vi "Word Report - Conditionally Formatted Table.vi"   [LabVIEW 2023]
doc: "This example shows how to format cells by their values in a Word document.\n\nThe VI sets the background color of the table cells to red if the cell value is greater than 90 and green if less than 10."
uses:
  <vilib>/Utility/NIReport.llb/Report Type.ctl
  <vilib>/Utility/NIReport.llb/NI_report.lvclass
  <vilib>/addons/_office/NI_ReportGenerationToolkit.lvlib
  <vilib>/Utility/NIReport.llb/Word/NI_Word.lvclass
  <vilib>/Utility/NIReport.llb/NI_ReportGenerationCore.lvlib
panel:
  # "Overview: This example shows how to format cells by their values. \nRequirements: Report Generation Toolkit, Microsoft Word\nInstructions:\nRun the VI.\n\nNote: Every Cell over the Value of 90 will be set to \"red\", if it is under the value of 10 it will be set to \"green\"."
types:
  T1 = typedef "NI_ReportGenerationCore.lvlib/Report Type.ctl" = enum16{"HTML", "Word", "Excel"}
  T2 = cluster{"Italic":enum16{"Italic Unchanged", "Italic On", "Italic Off"}, "Strike Through":enum16{"Strike Through Unchanged", "Strike Through On", "Strike Through Off"}, "Underline":enum16{"Underline Unchanged", "Underline On", "Underline Off"}, "Bold":enum16{"Bold Unchanged", "Bold On", "Bold Off"}}
  T3 = cluster{"OutsideLineStyle":i32, "OutsideColor":i32, "OutsideLineWidth":i32, "InsideLineStyle":i32, "InsideColor":i32, "InsideLineWidth":i32, "BackgroundPatternColor":i32}
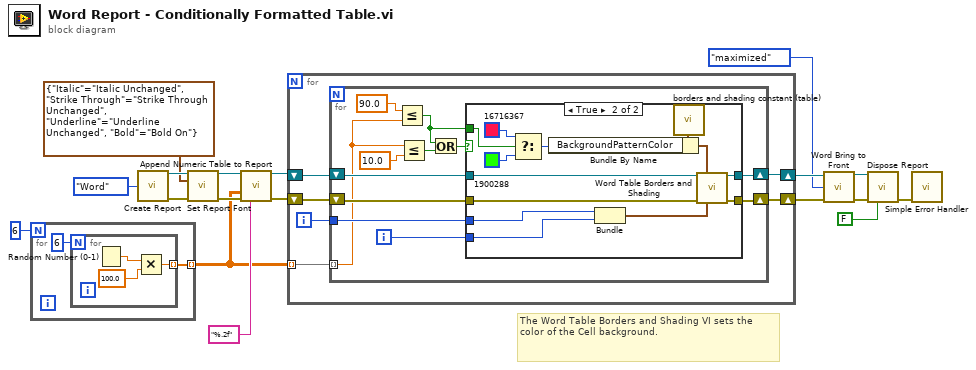
[diagram p0: block diagram]
diagram:
  # "The Word Table Borders and Shading VI sets the color of the Cell background."
  n1 = for {
    N: 6 -> [_]
    tunnel: [w19] -> w2 mode=indexing
    n2 = for {
      N: 6 ("dimension size") -> [_]
      tunnel: [w21] -> w19 mode=indexing
      n3 = Random Number (0-1)() -> (number: 0 to 1=w23:dbl)
      n4 = Multiply(x=w23, y=100.0) -> (x*y=w21:dbl)
    }
  }
  n5 = call <vilib>:"Create Report.vi"("report type"=Report_Type."Word" ("Report Type")) -> ("report out"=w14:refnum<class "NI_report.lvclass">, "error out"=w16:errorcluster)  [unwired: 13 in]
  n6 = call-dynamic "Set Report Font.vi"("report in"=w14, "text options"=T2 {"Italic"=enum."Italic Unchanged", "Strike Through"=enum."Strike Through Unchanged", "Underline"=enum."Underline Unchanged", "Bold"=enum."Bold On"}, "error in (no error)"=w16) -> ("report out"=w13:refnum<class "NI_report.lvclass">, "error out"=w15:errorcluster)  [unwired: 10 in, 1 out]
  n7 = call-dynamic "Append Numeric Table to Report.vi"("report in"=w13, "numerical data"=w2, "error in (no error)"=w15, "format string (%.3f)"="%.2f" ("format string")) -> ("report out"=w18:refnum<class "NI_report.lvclass">, "error out"=w17:errorcluster)  [unwired: 8 in, 2 out]
  n8 = for {
    shift-right: [w28] -> w9
    shift-left: w18 -> [w29]
    shift-right: [w26] -> w10
    shift-left: w17 -> [w27]
    tunnel: w2 -> [w24] mode=indexing
    i -> [w25]
    n9 = for {
      shift-right: [w40] -> w28
      shift-left: w29 -> [w39]
      shift-right: [w41] -> w26
      shift-left: w27 -> [w38]
      tunnel: w25 -> [w36]
      tunnel: w24 -> [w34] mode=indexing
      i -> [w30]
      n10 = Less Or Equal?(x=90.0 ("y"), y=w34) -> (x <= y?=w33:bool)
      n11 = Less Or Equal?(x=w34, y=10.0) -> (x <= y?=w32:bool)
      n12 = Or(x=w33, y=w32) -> (x .or. y?=w31:bool)
      n13 = case shown="True" w31 {
        tunnel: [w42 w56] -> w41
        tunnel: [w43 w55] -> w40
        tunnel: w30 -> [_ w44]
        tunnel: w36 -> [_ w45]
        tunnel: w39 -> [w43 w48]
        tunnel: w38 -> [w42 w47]
        tunnel: w33 -> [_ w46]
        frame False {
        }
        frame True {
          n14 = Select(t=u32 16716367, s=w46, f=u32 1900288) -> (s? t:f=w49:u32)
          n15 = Bundle(w45, w44) -> (w52:cluster{i32, i32})  [unwired: 1 in]
          n16 = call <vilib>:"borders and shading constant (table).vi"() -> ("borders and shading"=w54:T3)
          n17 = Bundle By Name(cluster=w54, "BackgroundPatternColor"=w49) -> (w53:T3)
          n18 = call <vilib>:"Word Table Borders and Shading.vi"("report in"=w48, "borders and shading"=w53, "error in (no error)"=w47, "start (-1, -1)"=w52) -> ("report out"=w55:refnum<class "NI_report.lvclass">, "error out"=w56:errorcluster)  [unwired: 10 in]
        }
      }
    }
  }
  n19 = call <vilib>:"Word Bring to Front.vi"("report in"=w9, "window state (maximized)"=enum16{"maximized", "minimized", "normal"}."maximized", "error in (no error)"=w10) -> ("report out"=w7:refnum<class "NI_report.lvclass">, "error out"=w6:errorcluster)  [unwired: 11 in]
  n20 = call-dynamic "Dispose Report.vi"("report in"=w7, "error in (no error)"=w6, "close report? (T)"=FALSE ("Close Report? (T)")) -> ("error out"=w5:errorcluster)  [unwired: 12 in]
  n21 = call <vilib>:"Simple Error Handler.vi"("error in (no error)"=w5) -> ()  [unwired: 4 in, 5 out]
